vi "Channel Info.vi"(8 "error in (no error)":errorcluster, 11 "Channel in":refnum<class "Channel.lvclass">) -> (0 "error out":errorcluster, 2 "Channel Info":T1, 3 "Channel out":refnum<class "Channel.lvclass">)   [LabVIEW 2020, in "VolatusConfig.lvlib" / "Channel.lvclass"]
uses:
  Channel.lvclass
  Channel.lvclass/Channel.ctl
  VolatusConfigElement/VolatusConfigElement.lvclass
  VolatusConfig.lvlib
  Meta Type.ctl
  lv-cdm/CDM-Config/Config Element/Config Element.lvclass
  lv-vecto/Vecto/Channel Info.ctl
  lv-vecto/VectoConfig/VectoConfig.lvlib
  C:/dev/lv20CE/relink/lv-volatus/VolatusConfig/VolatusConfigElement/VolatusConfigElement.lvclass
  C:/dev/lv20CE/relink/lv-volatus/VolatusConfig/Channel/Channel.lvclass
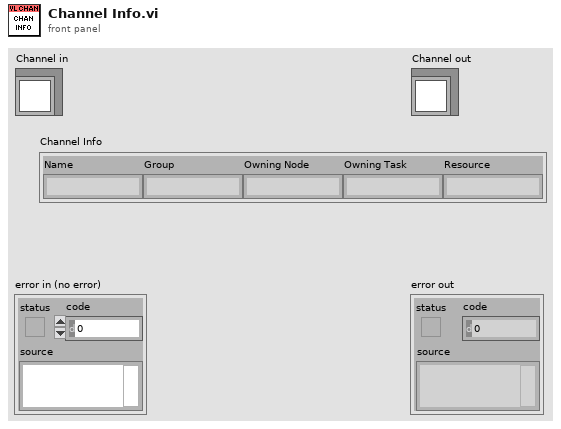
[diagram p1: front panel]
types:
  T1 = typedef "VectoConfig.lvlib/Channel Info.ctl" = cluster{"Name":string, "Group":string, "Owning Node":string, "Owning Task":string, "Resource":string}
  T2 = typedef "VolatusConfig.lvlib/Meta Type.ctl" = enum16{"UNKNOWN", "VL_System", "VL_Cluster", "VL_Node", "VL_Task", "VL_Group", "VL_Channel", "VL_Task_List", "VL_Scaling", "VL_Sensor", "VL_Sensor_List", "VL_Scale"}
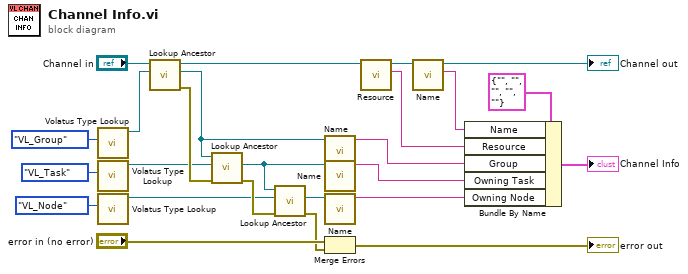
[diagram p0: block diagram]
diagram:
  n1 = call "Volatus Type Lookup.vi"("Meta Type"=Meta_Type."VL_Group") -> ("Config Lookup out"=w7:refnum<class "Config Lookup.lvclass">)  [unwired: 9 in, 1 out]
  n2 = call "Volatus Type Lookup.vi"("Meta Type"=Meta_Type."VL_Task") -> ("Config Lookup out"=w6:refnum<class "Config Lookup.lvclass">)  [unwired: 9 in, 1 out]
  n3 = call "Volatus Type Lookup.vi"("Meta Type"=Meta_Type."VL_Node") -> ("Config Lookup out"=w19:refnum<class "Config Lookup.lvclass">)  [unwired: 9 in, 1 out]
  n4 = call "Lookup Ancestor.vi"("Lookup"=w7, "VolatusConfigElement in"="Channel in") -> ("error out"=w24:errorcluster, "Ancestor"=w5:refnum<class "Config Element.lvclass">, "VolatusConfigElement out"=w11:refnum<class "Channel.lvclass">)  [unwired: 7 in]
  n5 = call "Lookup Ancestor.vi"("error in (no error)"=w24, "Lookup"=w6, "Config Element in"=w5) -> ("error out"=w25:errorcluster, "Ancestor"=w4:refnum<class "Config Element.lvclass">)  [unwired: 6 in, 1 out]
  n6 = call "Lookup Ancestor.vi"("error in (no error)"=w25, "Lookup"=w19, "Config Element in"=w4) -> ("error out"=w16:errorcluster, "Ancestor"=w18:refnum<class "Config Element.lvclass">)  [unwired: 6 in, 1 out]
  n7 = call "Name.vi"("Config Element in"=w5) -> ("Name"=w1:string)  [unwired: 9 in, 1 out]
  n8 = call "Name.vi"("Config Element in"=w4) -> ("Name"=w2:string)  [unwired: 9 in, 1 out]
  n9 = call "Name.vi"("Config Element in"=w18) -> ("Name"=w3:string)  [unwired: 9 in, 1 out]
  n10 = Merge Errors("error in (no error)", w16) -> (→"error out":errorcluster)
  n11 = call "Resource.vi"("Channel in"=w11) -> ("Resource"=w10:string, "Channel out"=w12:refnum<class "Channel.lvclass">)  [unwired: 8 in, 1 out]
  n12 = call "Name.vi"("VolatusConfigElement in"=w12) -> ("Name"=w13:string, "VolatusConfigElement out"=→"Channel out":refnum<class "Channel.lvclass">)  [unwired: 8 in, 1 out]
  n13 = Bundle By Name(cluster=T1 {"Name"="", "Group"="", "Owning Node"="", "Owning Task"="", "Resource"=""} ("Channel Info"), "Name"=w13, "Resource"=w10, "Group"=w1, "Owning Task"=w2, "Owning Node"=w3) -> (→"Channel Info":T1)
